vi "Update GUI frame rate.vi"(8 "error in (no error)":errorcluster, 11 "ImageStack in":refnum<class "ImageStack.lvclass">) -> (0 "error out":errorcluster, 3 "ImageStack out":refnum<class "ImageStack.lvclass">)   [LabVIEW 2012, in "ImageStack.lvclass"]
uses:
  ImageStack.lvclass
  ImageStack.lvclass/ImageStack.ctl
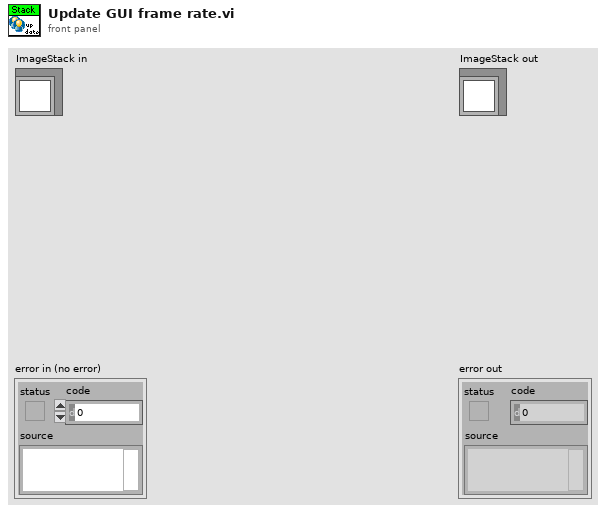
[diagram p1: front panel]
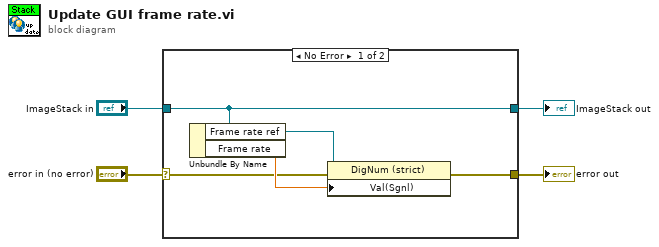
[diagram p0: block diagram]
diagram:
  n1 = case shown="No Error" "error in (no error)" {
    selector: "error in (no error)" -> [w6 w11]
    tunnel: [w5 w11] -> w3
    tunnel: [w9 w10] -> w1
    tunnel: "ImageStack in" -> [w9 w10]
    frame No Error {
      n2 = Unbundle By Name(w9) -> ("Frame rate ref"=w8:refnum<vi>, "Frame rate"=w7:dbl[unit])
      n3 = property class="DigNum (strict)"(reference=w8, error in=w6, "Val(Sgnl)"=w7) -> (error out=w5:errorcluster)  [unwired: 1 out]
    }
    frame Error {
    }
  }
  "error out" <- w3
  "ImageStack out" <- w1
